vi "PDC_GetDeviceName.vi"(8 "error in (no error)":errorcluster, 10 "ChildNo":u32, 11 "DeviceNo":u32) -> (0 "error out":errorcluster, 2 "StrName":string, 3 "ReturnValue":u32, 4 "ErrorCode":u32)   [LabVIEW 2015]
doc: "This VI retrieves the name of the specified device/child device."
uses:
  sub/global.vi
  PDCLIB.dll
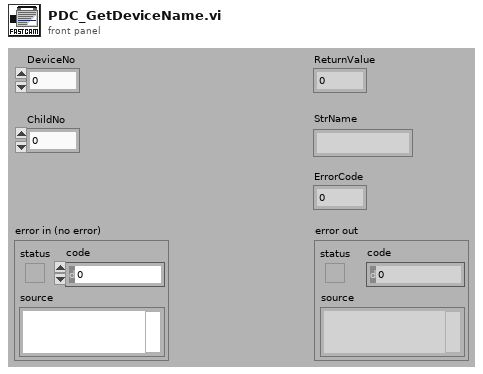
[diagram p1: front panel]
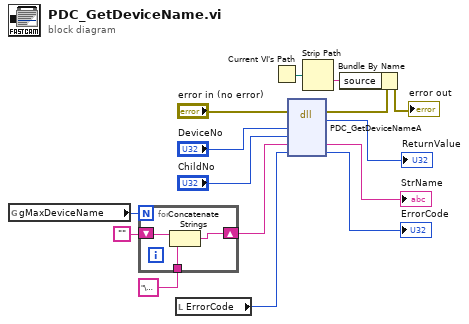
[diagram p0: block diagram]
diagram:
  n1 = global read "global.vi" "gMaxDeviceName"() -> (w5:i32)
  n2 = for {
    N: w5 -> [_]
    shift-right: [w18] -> w6
    shift-left: "" -> [w17]
    tunnel: "\u0000" -> [w16]
    n3 = Concatenate Strings(w17, w16) -> (w18:string)
  }
  n4 = local read "ErrorCode"() -> (w12:u32)
  n5 = Current VI's Path() -> (path=w3:path)
  n6 = dll-call lib="PDCLIB.dll" fn="PDC_GetDeviceNameA"(error in="error in (no error)", "nDeviceNo"="DeviceNo", "nChildNo"="ChildNo", "pStrName"=w6, "pErrorCode"=w12) -> (error out=w2:errorcluster, "return type"=→"ReturnValue":u32, "pStrName"=→"StrName":string, "pErrorCode"=→"ErrorCode":u32)  [unwired: 4 in, 1 out]
  n7 = Strip Path(path=w3) -> (name=w4:string)  [unwired: 1 out]
  n8 = Bundle By Name(cluster=w2, "source"=w4) -> (→"error out":errorcluster)
